vi "nn freemsg.vi"(8 "error in":errorcluster, 11 "message pointer":u64) -> (0 "error out":errorcluster)   [LabVIEW 2013, in "lvnano.lvlib"]
doc: "NN_EXPORT int nn_freemsg (void *msg);"
uses:
  lvnano.lvlib
  get last error code.vi
  get error string from code.vi
  <vilib>/Utility/error.llb/Error Cluster From Error Code.vi
  lvnanomsg.dll
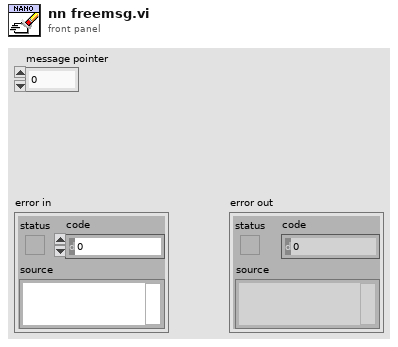
[diagram p1: front panel]
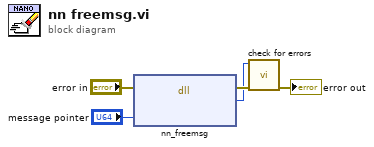
[diagram p0: block diagram]
diagram:
  n1 = dll-call lib="C:/Users/Daniel/Documents/nanomsg/lvnano/lvnanomsg.*" fn="nn_freemsg"(error in="error in", "message pointer"="message pointer") -> (error out=w3:errorcluster, "error"=w1:i32)  [unwired: 3 in, 1 out]
  n2 = call "check for errors.vi"("error in"=w3, "function return"=w1) -> ("error out"=→"error out":errorcluster)  [unwired: 9 in]
